vi "Add Additional Channels.vi"(8 "error in (no error)":errorcluster, 11 "Node Ptr":u64 format="%.0x") -> (0 "error out":errorcluster)   [LabVIEW 2010, in "PXIe-433x Custom Device.lvlib"]
uses:
  PXIe-433x Custom Device.lvlib
  Global.vi
  <vilib>/NI Veristand/Custom Device Tools/Custom Device Utility Library/NI VeriStand - Search for All Items by GUID.vi
  <vilib>/NI Veristand/Custom Device API/Custom Device API.lvlib
  <vilib>/NI Veristand/Custom Device Tools/Custom Device Utility Library/Custom Device Utility Library.lvlib
panel:
  in  "Tag":string
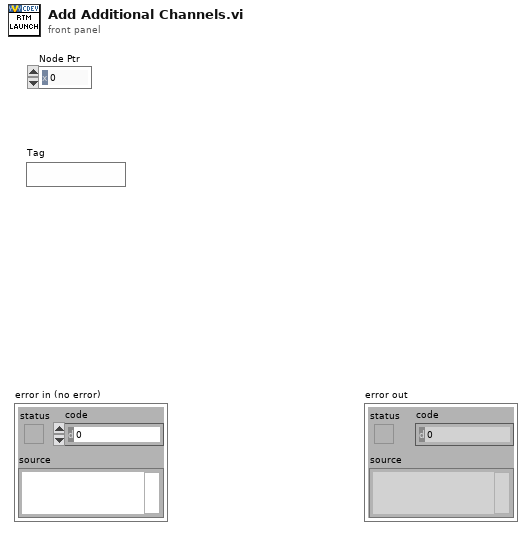
[diagram p1: front panel]
types:
  T1 = typedef "Custom Device API.lvlib/Custom Device Item Ref.ctl" = u64
  T2 = typedef "PXIe-433x Custom Device.lvlib/Max Value.ctl" = dbl
  T3 = typedef "PXIe-433x Custom Device.lvlib/Sensor Type.ctl" = enum16{"Strain", "Force", "Pressure", "Torque"}
  T4 = typedef "PXIe-433x Custom Device.lvlib/Min Value.ctl" = dbl
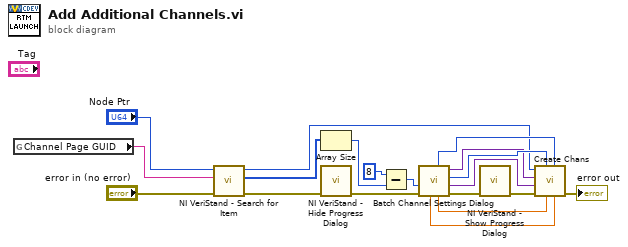
[diagram p0: block diagram]
diagram:
  n1 = global read "Global.vi" "Channel Page GUID"() -> (w10:string)
  n2 = call-poly <vilib>:"NI VeriStand - Search for Item.vi"("error in"="error in (no error)", "Item GUID"=w10, "Section Ref in"="Node Ptr") -> ("error out"=w6:errorcluster, "Item Refs"=w9:T1[], "Section Ref out"=w1:T1)  [unwired: 5 in, 1 out]
  n3 = Array Size(array=w9) -> (size(s)=w14:i32)
  n4 = call <vilib>:"NI VeriStand - Hide Progress Dialog.vi"("error in (no error)"=w6) -> ("error out"=w5:errorcluster)  [unwired: 10 in]
  n5 = Subtract(x=8, y=w14) -> (x-y=w19:i32)
  n6 = call "Batch Channel Settings Dialog.vi"("error in (no error)"=w5, "Data Entry Limits:Maximum"=w19) -> ("error out"=w4:errorcluster, "scaling information"=w12:variant, "# of Chans"=w16:u8, "bridge information"=w13:variant, "Maximum Value"=w18:T2, "Sensor Type"=w11:T3, "Minimum Value"=w17:T4)  [unwired: 3 in]
  n7 = call <vilib>:"NI VeriStand - Show Progress Dialog.vi"("error in (no error)"=w4) -> ("error out"=w3:errorcluster)  [unwired: 10 in]
  n8 = call "Create Chans.vi"("Minimum Value"=w17, "Sensor Type"=w11, "Maximum Value"=w18, "# of Chans"=w16, "error in"=w3, "scaling information"=w12, "bridge information"=w13, "Item Ref in"=w1) -> ("error out"=→"error out":errorcluster)  [unwired: 2 in, 1 out]
